vi "Get GUID.vi"(8 "error in (no error)":errorcluster caption="错误输入（无错误）", 11 "Item输入":refnum<class "Item.lvclass">) -> (0 "error out":errorcluster caption="错误输出", 2 "GUID":string, 3 "Item输出":refnum<class "Item.lvclass">)   [LabVIEW 2013, in "Hierarchy Framework.lvlib" / "Item.lvclass"]
uses:
  Item.lvclass
  Item.lvclass/Item.ctl
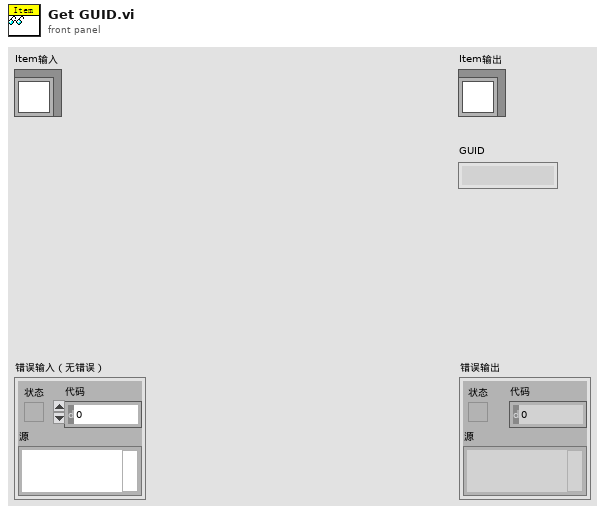
[diagram p1: front panel]
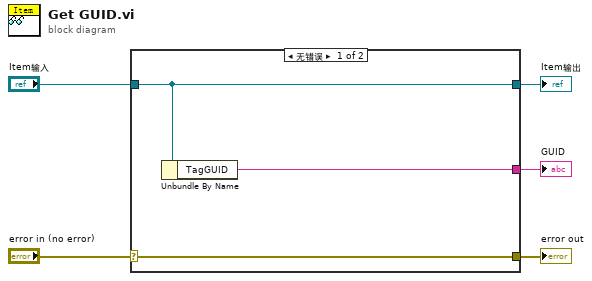
[diagram p0: block diagram]
diagram:
  n1 = case shown="无错误" "error in (no error)" {
    selector: "error in (no error)" -> [w8 w9]
    tunnel: [w8 w9] -> w4
    tunnel: [w7 w10] -> w2
    tunnel: "Item输入" -> [w7 w10]
    tunnel: [w6 _] -> w1
    frame No Error {
      n2 = Unbundle By Name(w7) -> ("TagGUID"=w6:string)
    }
    frame Error {
    }
  }
  "error out" <- w4
  "Item输出" <- w2
  "GUID" <- w1
